vi "SVT Gain and Phase (Frequency).vi"(0 "complex spectrum\nstimulus X":T9={"complex spectrum response"={"f0"=0.0, "df"=1.0, "complex spectrum"=[]}, "spectrum info"={"channel name"="", "description"="", "x-axis units"=0, "spectral info"={"spectrum type"=enum."Power [Magnitude^2]", "linear/dB"=enum."linear", "window"=0, "window size"=0, "FFT size"=0}, "engineering units"=0, "custom label"="", "dB reference [EU]"=0.0, "peak units"=enum."rms", "weighting filter"=0, "spectral density?"=FALSE, "unit label"="", "spectrum skewed?"=FALSE, "complimentary spectrum units"=enum."none"}} {"spectrum info"."x-axis units" items=["Time (s)"=0, "Frequency-CB (Hz)"=1, "Frequency-CPB (Hz)"=1248, "Frequency-Arbitrary (Hz)"=2357, "Quefrency (s)"=2, "Revolutions (rev)"=3, "Order"=4, "Speed (RPM)"=11, "Speed (rad/s)"=21, "Index"=65535]; "spectrum info"."weighting filter" items=["Linear", "A-weighting", "B-weighting", "C-weighting", "ITU-R 468-4", "Dolby", "CCITT", "C-message", "Wb", "Wc", "Wd", "We", "Wf", "Wh", "Wj", "Wk", "Wm", "AES17 20 kHz lowpass", "AES17 40 kHz lowpass", "AES17 20 kHz highpass", "AES17 40 kHz highpass"]; "spectrum info"."dB reference [EU]" format="%.2f"; "spectrum info"."engineering units" items=["custom..."=0, "V"=1, "A"=21, "C"=30, "pC"=31, "s"=32, "-"=29, "Pa"=2, "N"=20, "g"=3, "m/s^2"=4, "m/s"=5, "m"=6, "mm/s"=12, "mm"=13, "micron/s"=14, "micron"=15, "in/s^2"=7, "in/s"=8, "in"=9, "mil/s"=10, "mil"=11, "rad/s^2"=16, "rad/s"=17, "rad"=18, "deg/s^2"=26, "deg/s"=27, "deg"=28, "RPM"=22, "cycle/s^2"=23, "Hz"=24, "cycle"=25, "strain"=19]; "spectrum info"."spectral info"."window" items=["None "=0, "Hanning"=1, "Hamming"=2, "Blackman-Harris"=3, "Exact Blackman"=4, "Blackman"=5, "Flat Top"=6, "4 Term B-Harris "=7, "7 Term B-Harris"=8, "Low Sidelobe"=9, "Force - Exponential"=10, "Gaussian"=62]; "complex spectrum response"."complex spectrum" format="%.2f"; "complex spectrum response"."df" format="%.2f"; "complex spectrum response"."f0" format="%.2f"}, 1 "complex spectrum\nresponse Y":T9={"complex spectrum response"={"f0"=0.0, "df"=1.0, "complex spectrum"=[]}, "spectrum info"={"channel name"="", "description"="", "x-axis units"=0, "spectral info"={"spectrum type"=enum."Power [Magnitude^2]", "linear/dB"=enum."linear", "window"=0, "window size"=0, "FFT size"=0}, "engineering units"=0, "custom label"="", "dB reference [EU]"=0.0, "peak units"=enum."rms", "weighting filter"=0, "spectral density?"=FALSE, "unit label"="", "spectrum skewed?"=FALSE, "complimentary spectrum units"=enum."none"}} {"spectrum info"."x-axis units" items=["Time (s)"=0, "Frequency-CB (Hz)"=1, "Frequency-CPB (Hz)"=1248, "Frequency-Arbitrary (Hz)"=2357, "Quefrency (s)"=2, "Revolutions (rev)"=3, "Order"=4, "Speed (RPM)"=11, "Speed (rad/s)"=21, "Index"=65535]; "spectrum info"."weighting filter" items=["Linear", "A-weighting", "B-weighting", "C-weighting", "ITU-R 468-4", "Dolby", "CCITT", "C-message", "Wb", "Wc", "Wd", "We", "Wf", "Wh", "Wj", "Wk", "Wm", "AES17 20 kHz lowpass", "AES17 40 kHz lowpass", "AES17 20 kHz highpass", "AES17 40 kHz highpass"]; "spectrum info"."dB reference [EU]" format="%.2f"; "spectrum info"."engineering units" items=["custom..."=0, "V"=1, "A"=21, "C"=30, "pC"=31, "s"=32, "-"=29, "Pa"=2, "N"=20, "g"=3, "m/s^2"=4, "m/s"=5, "m"=6, "mm/s"=12, "mm"=13, "micron/s"=14, "micron"=15, "in/s^2"=7, "in/s"=8, "in"=9, "mil/s"=10, "mil"=11, "rad/s^2"=16, "rad/s"=17, "rad"=18, "deg/s^2"=26, "deg/s"=27, "deg"=28, "RPM"=22, "cycle/s^2"=23, "Hz"=24, "cycle"=25, "strain"=19]; "spectrum info"."spectral info"."window" items=["None "=0, "Hanning"=1, "Hamming"=2, "Blackman-Harris"=3, "Exact Blackman"=4, "Blackman"=5, "Flat Top"=6, "4 Term B-Harris "=7, "7 Term B-Harris"=8, "Low Sidelobe"=9, "Force - Exponential"=10, "Gaussian"=62]; "complex spectrum response"."complex spectrum" format="%.2f"; "complex spectrum response"."df" format="%.2f"; "complex spectrum response"."f0" format="%.2f"}, 3 "advanced span [Hz]":dbl=-1.0 format="%.2f", 5 "error in (no error)":errorcluster, 6 "desired units":T2, 9 "expected fundamental frequency [Hz]":dbl=-1.0 format="%.2f") -> (11 "detected tone response":cluster{"frequency [Hz]":dbl, "amplitude":dbl}={"frequency [Hz]"=nan, "amplitude"=nan} {"amplitude" format="%.3f"; "frequency [Hz]" format="%.2f"}, 12 "unit labels":T1, 13 "detected tone stimulus":cluster{"frequency [Hz]":dbl, "amplitude":dbl}={"frequency [Hz]"=nan, "amplitude"=nan} {"amplitude" format="%.3f"; "frequency [Hz]" format="%.2f"}, 14 "dup complex spectrum\nstimulus X":T9={"complex spectrum response"={"f0"=0.0, "df"=1.0, "complex spectrum"=[]}, "spectrum info"={"channel name"="", "description"="", "x-axis units"=0, "spectral info"={"spectrum type"=enum."Power [Magnitude^2]", "linear/dB"=enum."linear", "window"=0, "window size"=0, "FFT size"=0}, "engineering units"=0, "custom label"="", "dB reference [EU]"=0.0, "peak units"=enum."rms", "weighting filter"=0, "spectral density?"=FALSE, "unit label"="", "spectrum skewed?"=FALSE, "complimentary spectrum units"=enum."none"}} {"spectrum info"."x-axis units" items=["Time (s)"=0, "Frequency-CB (Hz)"=1, "Frequency-CPB (Hz)"=1248, "Frequency-Arbitrary (Hz)"=2357, "Quefrency (s)"=2, "Revolutions (rev)"=3, "Order"=4, "Speed (RPM)"=11, "Speed (rad/s)"=21, "Index"=65535]; "spectrum info"."weighting filter" items=["Linear", "A-weighting", "B-weighting", "C-weighting", "ITU-R 468-4", "Dolby", "CCITT", "C-message", "Wb", "Wc", "Wd", "We", "Wf", "Wh", "Wj", "Wk", "Wm", "AES17 20 kHz lowpass", "AES17 40 kHz lowpass", "AES17 20 kHz highpass", "AES17 40 kHz highpass"]; "spectrum info"."dB reference [EU]" format="%.2f"; "spectrum info"."engineering units" items=["custom..."=0, "V"=1, "A"=21, "C"=30, "pC"=31, "s"=32, "-"=29, "Pa"=2, "N"=20, "g"=3, "m/s^2"=4, "m/s"=5, "m"=6, "mm/s"=12, "mm"=13, "micron/s"=14, "micron"=15, "in/s^2"=7, "in/s"=8, "in"=9, "mil/s"=10, "mil"=11, "rad/s^2"=16, "rad/s"=17, "rad"=18, "deg/s^2"=26, "deg/s"=27, "deg"=28, "RPM"=22, "cycle/s^2"=23, "Hz"=24, "cycle"=25, "strain"=19]; "spectrum info"."spectral info"."window" items=["None "=0, "Hanning"=1, "Hamming"=2, "Blackman-Harris"=3, "Exact Blackman"=4, "Blackman"=5, "Flat Top"=6, "4 Term B-Harris "=7, "7 Term B-Harris"=8, "Low Sidelobe"=9, "Force - Exponential"=10, "Gaussian"=62]; "complex spectrum response"."complex spectrum" format="%.2f"; "complex spectrum response"."df" format="%.2f"; "complex spectrum response"."f0" format="%.2f"}, 15 "dup complex spectrum\nresponse Y":T9={"complex spectrum response"={"f0"=0.0, "df"=1.0, "complex spectrum"=[]}, "spectrum info"={"channel name"="", "description"="", "x-axis units"=0, "spectral info"={"spectrum type"=enum."Power [Magnitude^2]", "linear/dB"=enum."linear", "window"=0, "window size"=0, "FFT size"=0}, "engineering units"=0, "custom label"="", "dB reference [EU]"=0.0, "peak units"=enum."rms", "weighting filter"=0, "spectral density?"=FALSE, "unit label"="", "spectrum skewed?"=FALSE, "complimentary spectrum units"=enum."none"}} {"spectrum info"."x-axis units" items=["Time (s)"=0, "Frequency-CB (Hz)"=1, "Frequency-CPB (Hz)"=1248, "Frequency-Arbitrary (Hz)"=2357, "Quefrency (s)"=2, "Revolutions (rev)"=3, "Order"=4, "Speed (RPM)"=11, "Speed (rad/s)"=21, "Index"=65535]; "spectrum info"."weighting filter" items=["Linear", "A-weighting", "B-weighting", "C-weighting", "ITU-R 468-4", "Dolby", "CCITT", "C-message", "Wb", "Wc", "Wd", "We", "Wf", "Wh", "Wj", "Wk", "Wm", "AES17 20 kHz lowpass", "AES17 40 kHz lowpass", "AES17 20 kHz highpass", "AES17 40 kHz highpass"]; "spectrum info"."dB reference [EU]" format="%.2f"; "spectrum info"."engineering units" items=["custom..."=0, "V"=1, "A"=21, "C"=30, "pC"=31, "s"=32, "-"=29, "Pa"=2, "N"=20, "g"=3, "m/s^2"=4, "m/s"=5, "m"=6, "mm/s"=12, "mm"=13, "micron/s"=14, "micron"=15, "in/s^2"=7, "in/s"=8, "in"=9, "mil/s"=10, "mil"=11, "rad/s^2"=16, "rad/s"=17, "rad"=18, "deg/s^2"=26, "deg/s"=27, "deg"=28, "RPM"=22, "cycle/s^2"=23, "Hz"=24, "cycle"=25, "strain"=19]; "spectrum info"."spectral info"."window" items=["None "=0, "Hanning"=1, "Hamming"=2, "Blackman-Harris"=3, "Exact Blackman"=4, "Blackman"=5, "Flat Top"=6, "4 Term B-Harris "=7, "7 Term B-Harris"=8, "Low Sidelobe"=9, "Force - Exponential"=10, "Gaussian"=62]; "complex spectrum response"."complex spectrum" format="%.2f"; "complex spectrum response"."df" format="%.2f"; "complex spectrum response"."f0" format="%.2f"}, 16 "gain":dbl=nan format="%.2f", 17 "phase lag":dbl=nan format="%.2f", 19 "error out":errorcluster)   [LabVIEW 2017, in "SoundVib_SingleTone.lvlib"]
doc: "Computes the gain and phase between <B>stimulus signal X</B> and <B>response signal Y</B> at the fundamental frequency. This VI returns the detected fundamental frequency, detected response amplitude, gain, and phase lag. This VI does not maintain state internally; you can use this VI in a loop to process multiple blocks. Wire data to the <B>stimulus signal X [Eux]</B> and <B>response signal Y [Euy]</B> inputs to determine the polymorphic instance to use or manually select the instance."
uses:
  <vilib>/addons/Sound and Vibration/svt_Single Tone Measurements/SoundVib_SingleTone.lvlib
  <vilib>/addons/_NISVFA/_Shared subVIs/Controls/svc_Spectrum Info.ctl
  <vilib>/addons/_NISVFA/_Shared subVIs/Controls/svc_X-Axis Units.ctl
  <vilib>/addons/_NISVFA/_Shared subVIs/Controls/svc_Spectrum Type.ctl
  <vilib>/addons/_NISVFA/_Shared subVIs/Controls/svc_Engineering Units Text Ring.ctl
  <vilib>/addons/_NISVFA/_Shared subVIs/Controls/svc_Weighting Filter Text Ring.ctl
  <vilib>/addons/_NISVFA/_Shared subVIs/Controls/svc_Complimentary Spectrum Units.ctl
  <vilib>/addons/_NISVFA/_Spectrum Processing/SVFA Get Spectrum Value (1 Ch).vi
  <vilib>/addons/_NISVFA/_Shared subVIs/Common/svc_Spectrum Units.vi
  <vilib>/addons/_NISVFA/_Shared subVIs/Common/svc_Convert Frequency to Frequency String.vi
  <vilib>/addons/_NISVFA/_Shared subVIs/Common/svc_Get Weighting Enum and Labels.vi
  <vilib>/addons/_NISVFA/_Shared subVIs/Common/svc_Unit Label Lexical Class.vi
  <vilib>/addons/_NISVFA/_Shared subVIs/Common/svc_Engineering Units to Unit Label.vi
  <vilib>/addons/_NISVFA/_Shared subVIs/Common/svc_Format Value (DBL).vi
  <vilib>/addons/_NISVFA/_Spectrum Processing/SVFA Unit Conversion (Complex) (1 Ch).vi
  <vilib>/addons/Sound and Vibration/svt_Distortion/SoundVib_Distortion.lvlib
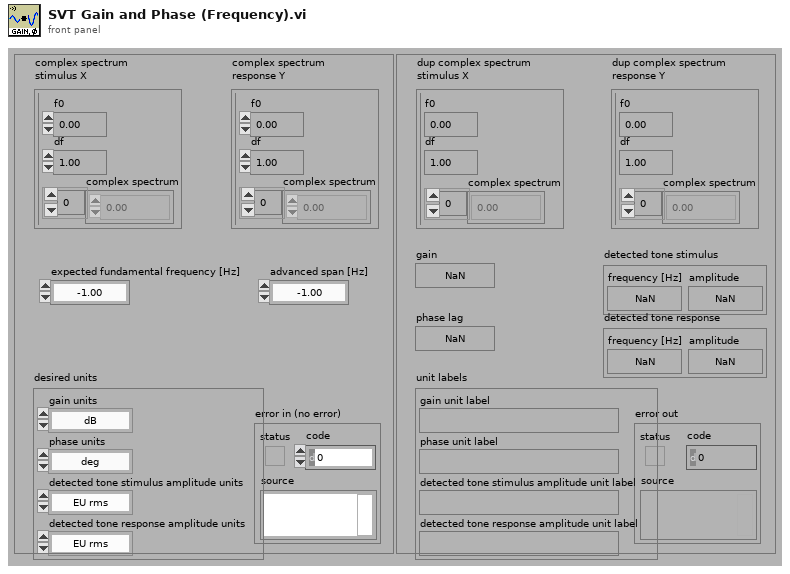
[diagram p1: front panel]
types:
  T1 = cluster{"gain unit label":string, "phase unit label":string, "detected tone stimulus amplitude unit label":string, "detected tone response amplitude unit label":string}
  T2 = cluster{"gain units":enum16{"dB", "linear ratio"}, "phase units":enum16{"deg", "rad"}, "detected tone stimulus amplitude units":enum16{"EU rms", "EU peak", "EU peak-peak"}, "detected tone response amplitude units":enum16{"EU rms", "EU peak", "EU peak-peak"}}
  T3 = typedef "svc_Spectrum Info.ctl" = cluster{"channel name":string, "description":string, "x-axis units":T4, "spectral info":cluster{"spectrum type":T5, "linear/dB":enum16{"linear", "dB"}, "window":u16, "window size":i32, "FFT size":i32}, "engineering units":T6, "custom label":string, "dB reference [EU]":dbl, "peak units":enum16{"rms", "peak", "peak-peak"}, "weighting filter":T7, "spectral density?":bool, "unit label":string, "spectrum skewed?":bool, "complimentary spectrum units":T8}
  T4 = typedef "svc_X-Axis Units.ctl" = u16
  T5 = typedef "svc_Spectrum Type.ctl" = enum16{"FFT Spectrum [complex]", "Amplitude [Magnitude]", "Power [Magnitude^2]", "Cross Spectrum [complex]", "Frequency Response [Complex]"}
  T6 = typedef "svc_Engineering Units Text Ring.ctl" = u16
  T7 = typedef "svc_Weighting Filter Text Ring.ctl" = u16
  T8 = typedef "svc_Complimentary Spectrum Units.ctl" = enum16{"none", "radians", "degrees", "cycles", "imaginary"}
  T9 = cluster{"complex spectrum response":cluster{"f0":dbl, "df":dbl, "complex spectrum":cdb[]}, "spectrum info":T3}
  T10 = enum32{"none", "input signal", "detected signal", "residual signal"}
  T11 = cluster{"gain":string, "phase":string, "stim. a":string, "resp. a":string}
  T12 = enum16{"coerce to nearest", "coerce to next highest", "coerce to next lowest", "interpolate"}
  T13 = cluster{"linear/dB":enum16{"no change", "linear", "dB"}, "dB reference (0: no change)":dbl, "power/magnitude":enum16{"no change", "power", "magnitude"}, "view":enum16{"no change", "rms", "peak", "peak-peak"}}
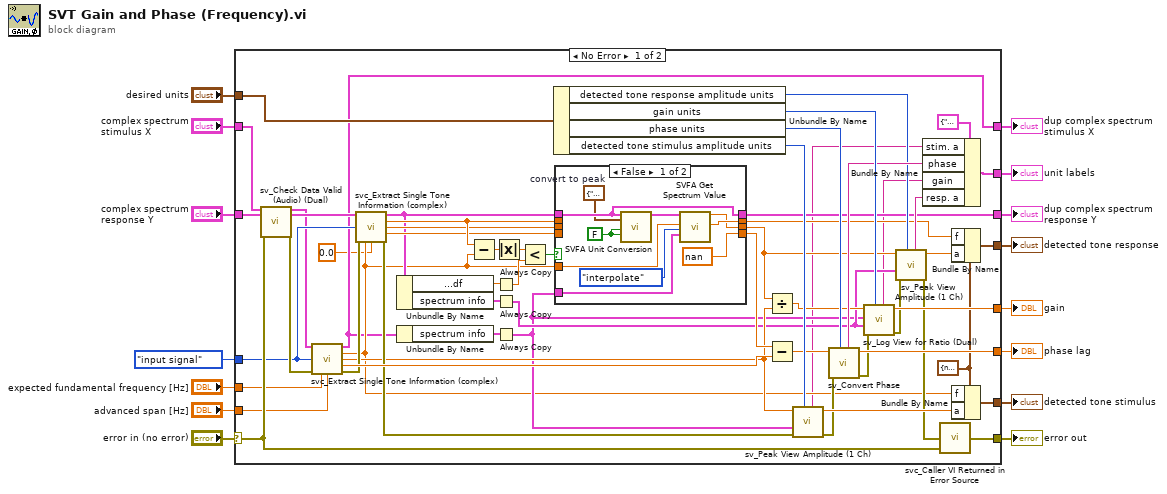
[diagram p0: block diagram]
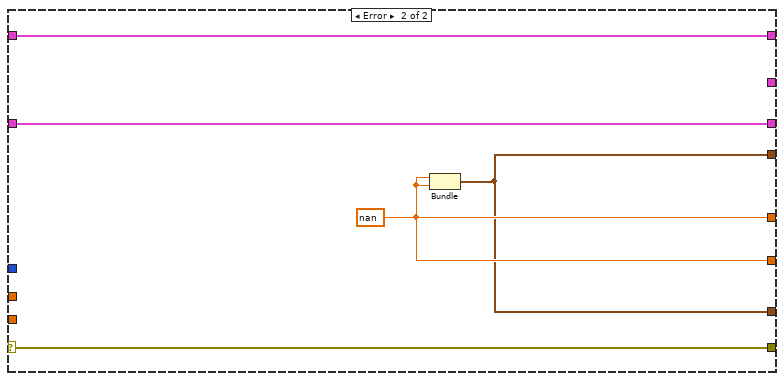
[diagram p3: hidden frame]
diagram:
  n1 = case shown="No Error" "error in (no error)" {
    selector: "error in (no error)" -> [w60 w92]
    tunnel: "complex spectrum\nresponse Y" -> [w65 w91]
    tunnel: [w68 w89] -> w14
    tunnel: [w66 w92] -> w13
    tunnel: "complex spectrum\nstimulus X" -> [w64 w90]
    tunnel: [w69 w89] -> w11
    tunnel: [w73 w88] -> w9
    tunnel: [w72 w88] -> w8
    tunnel: "desired units" -> [w71 _]
    tunnel: [w67 _] -> w6
    tunnel: [w31 w91] -> w5
    tunnel: [w19 w90] -> w4
    tunnel: T10."input signal" ("export signals") -> [w30 _]
    tunnel: "expected fundamental frequency [Hz]" -> [w17 _]
    tunnel: "advanced span [Hz]" -> [w18 _]
    frame No Error {
      w23 = cluster{"f":dbl, "a":dbl} {"f"=nan, "a"=nan} ("detected tone stimulus")
      n2 = call <vilib>:"sv_Check Data Valid (Audio) (Dual).vi"("complex spectrum stimulus"=w64, "complex spectrum response"=w65, "error in (no error)"=w60) -> (14:"complex spectrum"=w27:T9, 15:"complex spectrum"=w61:T9, "error out"=w63:errorcluster)  [unwired: 14 in]
      n3 = call <vilib>:"svc_Extract Single Tone Information (complex).vi"("complex spectrum"=w27, "export signals"=w30, "error in"=w63, "approximate frequency [Hz]"=w17, "advanced span [Hz]"=w18) -> ("complex spectrum"=w19:T9, "frequency [Hz]"=w24:dbl, "amplitude [EU pk]"=w29:dbl, "phase [deg]"=w62:dbl, "error out"=w55:errorcluster)  [unwired: 5 in, 1 out]
      n4 = call <vilib>:"svc_Extract Single Tone Information (complex).vi"("complex spectrum"=w61, "export signals"=w30, "error in"=w55, "approximate frequency [Hz]"=w24, "advanced span [Hz]"=0.0) -> ("complex spectrum"=w28:T9, "frequency [Hz]"=w43:dbl, "amplitude [EU pk]"=w41:dbl, "phase [deg]"=w39:dbl, "error out"=w54:errorcluster)  [unwired: 5 in, 1 out]
      n5 = Unbundle By Name(w28) -> ("complex spectrum response.df"=w45:dbl, "spectrum info"=w34:T3)
      n6 = Unbundle By Name(w19) -> ("spectrum info"=w44:T3)
      n7 = Subtract(x=w43, y=w24) -> (x-y=w57:dbl)
      n8 = Always Copy(1:w45) -> (0:w33:dbl)
      n9 = Always Copy(1:w34) -> (0:w26:T3)
      n10 = Always Copy(1:w44) -> (0:w25:T3)
      n11 = Absolute Value(x=w57) -> (abs(x)=w56:dbl)
      n12 = Less?(x=w56, y=w33) -> (x < y?=w46:bool)
      n13 = Unbundle By Name(w71) -> ("detected tone response amplitude units"=w51:enum16{"EU rms", "EU peak", "EU peak-peak"}, "gain units"=w59:enum16{"dB", "linear ratio"}, "phase units"=w53:enum16{"deg", "rad"}, "detected tone stimulus amplitude units"=w52:enum16{"EU rms", "EU peak", "EU peak-peak"})
      n14 = case shown="False" w46 {
        tunnel: w28 -> [w75 w84]
        tunnel: w24 -> [w81 _]
        tunnel: w25 -> [w79 _]
        tunnel: w43 -> [_ w87]
        tunnel: [w78 w87] -> w42
        tunnel: w41 -> [_ w86]
        tunnel: [w77 w86] -> w40
        tunnel: w39 -> [_ w85]
        tunnel: [nan ("detected phase (deg)") w85] -> w38
        tunnel: [w75 w84] -> w31
        frame False {
          w74 = T13 {"linear/dB"=enum."no change", "dB reference (0: no change)"=0.0, "power/magnitude"=enum."no change", "view"=enum."peak"}  # convert to peak
          w83 = FALSE ("convert to degree (T)")
          n15 = call-poly <vilib>:"SVFA Unit Conversion.vi"("complex spectrum"=w75, "desired scaling"=w74, "unwrap phase (F)"=w83, "convert to degree (T)"=w83) -> ("converted spectrum"=w82:cluster{"x0":dbl, "dx":dbl, "magnitude":dbl[]})  [unwired: 10 in, 5 out]
          n16 = call-poly <vilib>:"SVFA Get Spectrum Value.vi"("spectrum"=w82, "x value (1000)"=w81, "coercion (nearest)"=T12."interpolate" ("frequency coercion"), "spectrum info"=w79) -> ("spectrum value"=w77:dbl, "actual x value"=w78:dbl)  [unwired: 11 in, 3 out]
        }
        frame True {
        }
      }
      n17 = Divide(x=w40, y=w29) -> (x/y=w48:dbl)
      n18 = Subtract(x=w38, y=w62) -> (x-y=w47:dbl)
      n19 = call <vilib>:"sv_Peak View Amplitude (1 Ch).vi"("peak units"=w52, "error in (no error)"=w54, "spectrum info"=w25, "peak amplitude [EU pk]"=w29) -> ("error out"=w36:errorcluster, "converted peak amplitude"=w70:dbl, "unit label"=w21:string)  [unwired: 5 in]
      n20 = call <vilib>:"sv_Convert Phase.vi"("phase units"=w53, "error in (no error)"=w36, "phase lag [deg]"=w47) -> ("error out"=w37:errorcluster, "converted phase lag"=w68:dbl, "phase unit label"=w58:string)  [unwired: 6 in]
      n21 = call <vilib>:"sv_Log View for Ratio (Dual).vi"("ratio units"=w59, "error in (no error)"=w37, "spectrum info Y"=w26, "spectrum info X"=w25, "linear ratio (Y/X)"=w48) -> ("error out"=w35:errorcluster, "converted ratio"=w69:dbl, "unit label"=w20:string)  [unwired: 4 in]
      n22 = call <vilib>:"sv_Peak View Amplitude (1 Ch).vi"("peak units"=w51, "error in (no error)"=w35, "spectrum info"=w26, "peak amplitude [EU pk]"=w40) -> ("error out"=w32:errorcluster, "converted peak amplitude"=w50:dbl, "unit label"=w49:string)  [unwired: 5 in]
      n23 = Bundle By Name(cluster=T11 {"gain"="", "phase"="", "stim. a"="", "resp. a"=""} ("unit labels"), "stim. a"=w21, "phase"=w58, "gain"=w20, "resp. a"=w49) -> (w67:T11)
      n24 = call <vilib>:"svc_Caller VI Returned in Error Source.vi"("warning input to caller"=w60, "error in (no error)"=w32) -> ("error out"=w66:errorcluster)  [unwired: 3 in]
      n25 = Bundle By Name(cluster=w23, "f"=w42, "a"=w50) -> (w73:cluster{"f":dbl, "a":dbl})
      n26 = Bundle By Name(cluster=w23, "f"=w24, "a"=w70) -> (w72:cluster{"f":dbl, "a":dbl})
    }
    frame Error {
      w89 = nan
      n27 = Bundle(w89, w89) -> (w88:cluster{dbl, dbl})  [unwired: 1 in]
    }
  }
  "phase lag" <- w14
  "error out" <- w13
  "gain" <- w11
  "dup complex spectrum\nresponse Y" <- w5
  "dup complex spectrum\nstimulus X" <- w4
  "unit labels" <- w6
  "detected tone response" <- w9
  "detected tone stimulus" <- w8
